vi "LB_ItemName_Tests.vi"(11 "error in":errorcluster) -> (15 "error out":errorcluster)   [LabVIEW 2016, in "DronaTest.lvlib"]
uses:
  DronaTest.lvlib
  APIs/Stimulus/ControlValue/SetValueAuto.vi
  APIs/Stimulus/ControlValue/Controls/Listbox/SetValueByItemName.vi
  APIs/Assert/AssertControlValue/Equal.vi
  <vilib>/addons/_JKI Toolkits/Caraya/classes/Assert/Assert Equal Value_Variant.vi
  <vilib>/addons/_JKI Toolkits/Caraya/classes/Assert/Assert Error.vi
  <vilib>/addons/_JKI Toolkits/Caraya/classes/Test/Test.lvclass
  Drona.lvlib
  <vilib>/SLL Toolkit/SLL Debug/SLL Debug.lvlib
  APIs/Assert/AssertControlValue/AssertControlValue.lvlib
  APIs/Stimulus/ControlValue/ControlValue.lvlib
  <vilib>/addons/_JKI Toolkits/Caraya/classes/Assert/Assert.lvclass
  APIs/Stimulus/ControlValue/Controls/Listbox/StimulusListbox.lvlib
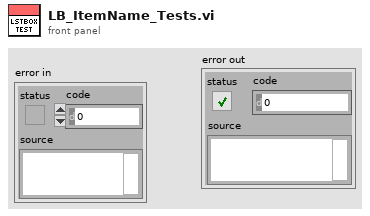
[diagram p1: front panel]
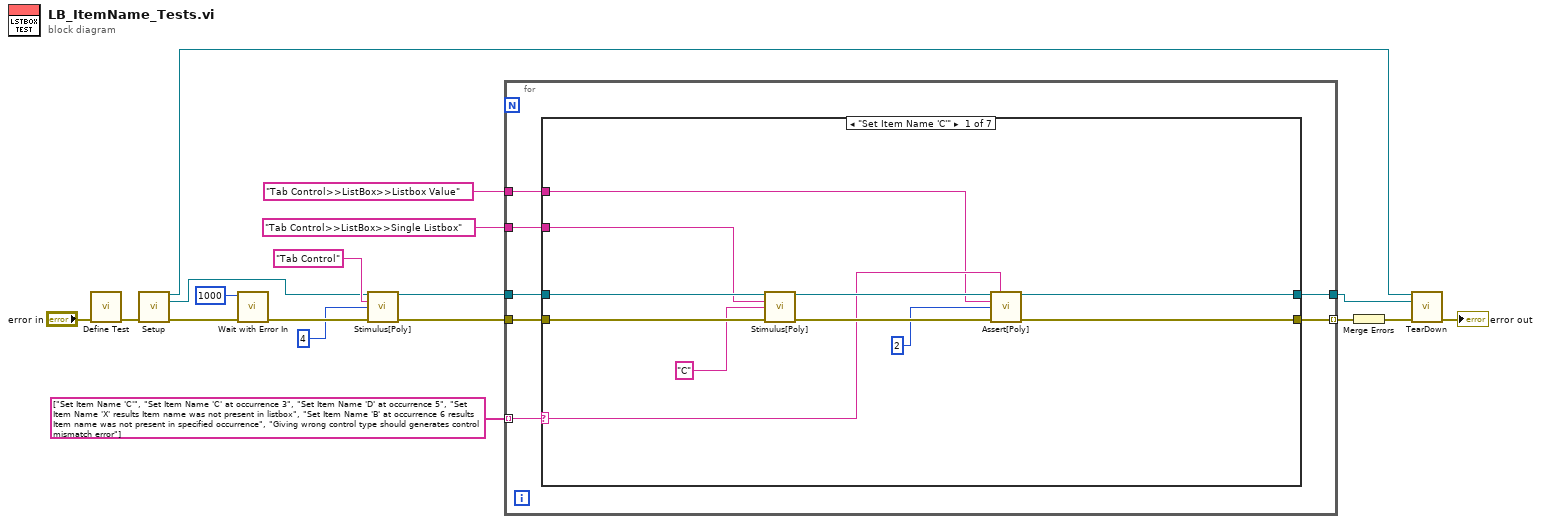
[diagram p0: block diagram]
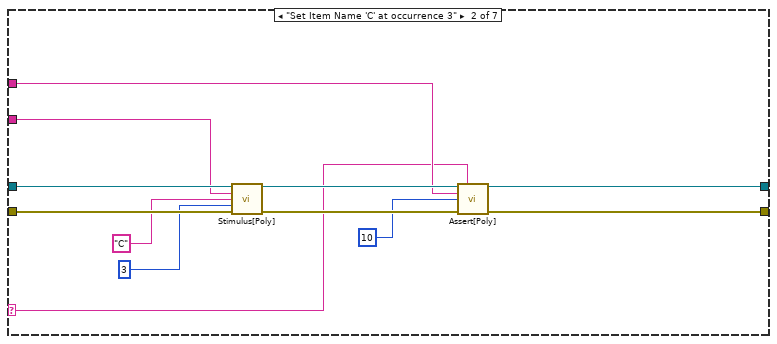
[diagram p2: hidden frame]
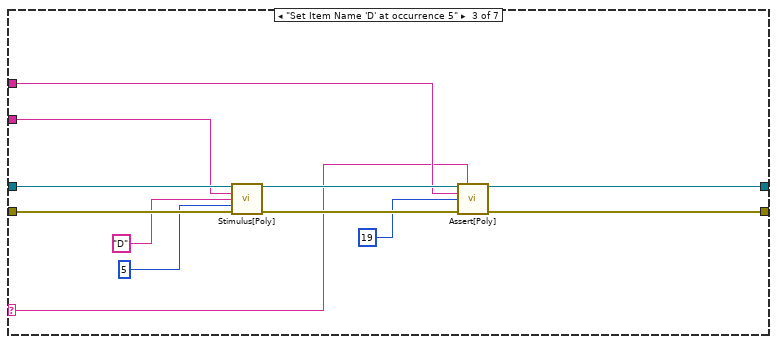
[diagram p3: hidden frame]
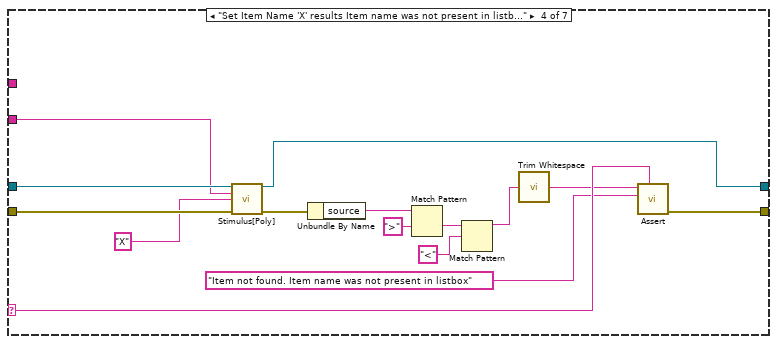
[diagram p4: hidden frame]
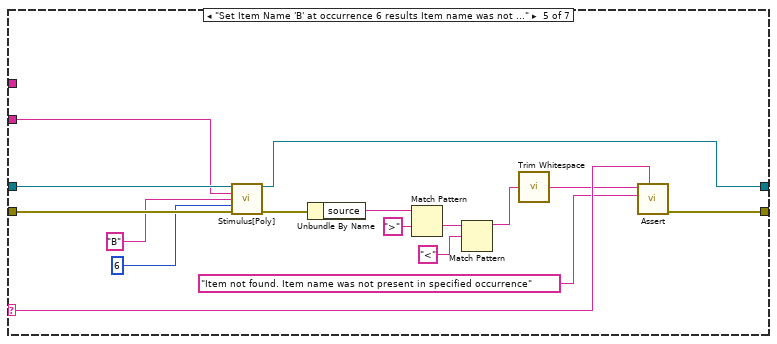
[diagram p5: hidden frame]
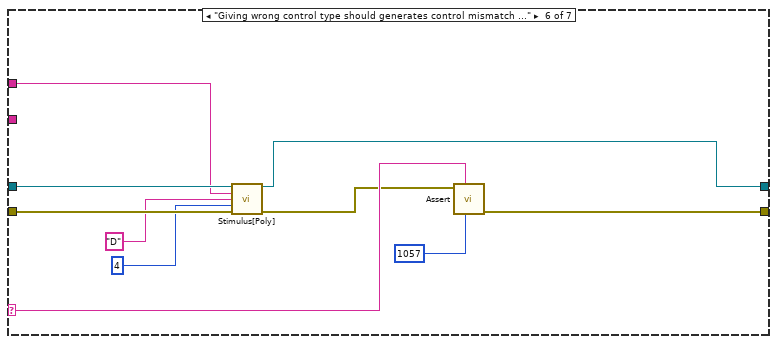
[diagram p6: hidden frame]
diagram:
  n1 = call <vilib>:"Define Test.vi"("error in (no error)"="error in") -> ("error out"=w7:errorcluster)  [unwired: 10 in]
  n2 = call "Setup.vi"("error in (no error)"=w7) -> ("Application Ref"=w2:refnum<vi>, "VI out"=w6:refnum<vi>, "error out"=w5:errorcluster)  [unwired: 12 in]
  n3 = call <vilib>:"Wait with Error In.vi"("error in (no error)"=w5, "milliseconds to wait"=u32 1000) -> ("error out"=w16:errorcluster)  [unwired: 9 in]
  n4 = call-poly "Stimulus[Poly].vi"("VI Reference In"=w6, "Control Path"="Tab Control", "Value (Signaling)"=4, "error in"=w16) -> ("VI Reference Out"=w12:refnum<vi>, "error out"=w15:errorcluster)  [unwired: 10 in]
  n5 = for {
    tunnel: w12 -> [w24]
    tunnel: "Tab Control>>ListBox>>Single Listbox" ("Control Path") -> [w23]
    tunnel: "Tab Control>>ListBox>>Listbox Value" ("Control Path") -> [w22]
    tunnel: string[] ["Set Item Name 'C'", "Set Item Name 'C' at occurrence 3", "Set Item Name 'D' at occurrence 5", "Set Item Name 'X' results Item name was not present in listbox", "Set Item Name 'B' at occurrence 6 results Item name was not present in specified occurrence", "Giving wrong control type should generates control mismatch error"] -> [w20] mode=indexing
    tunnel: [w19] -> w3
    tunnel: w15 -> [w25]
    tunnel: [w21] -> w8 mode=indexing
    n6 = case shown="\"Set Item Name 'C'\"" w20 {
      selector: w20 -> [w30 w40 w52 w71 w87 w98 _]
      tunnel: w25 -> [w36 w48 w60 w75 w91 w101 w103]
      tunnel: w24 -> [w35 w47 w59 w74 w90 w100 w102]
      tunnel: w23 -> [w26 w44 w56 w73 w89 _ _]
      tunnel: w22 -> [w27 w43 w55 _ _ w92 _]
      tunnel: [w32 w42 w54 w72 w88 w99 w103] -> w21
      tunnel: [w31 w41 w53 w70 w86 w97 w102] -> w19
      frame "Set Item Name 'C'" {
        n7 = call-poly "Stimulus[Poly].vi"("VI Reference In"=w35, "Control Path"=w26, "Item Name"="C", "Error In"=w36) -> ("VI Reference Out"=w33:refnum<vi>, "Error Out"=w34:errorcluster)  [unwired: 10 in]
        n8 = call-poly "Assert[Poly].vi"("VI Reference In"=w33, "Test Label"=w30, "Control Path"=w27, "Control Value"=2, "Error In"=w34) -> ("VI Reference Out"=w31:refnum<vi>, "Error Out"=w32:errorcluster)  [unwired: 8 in, 1 out]
      }
      frame "Set Item Name 'C' at occurrence 3" {
        n9 = call-poly "Stimulus[Poly].vi"("VI Reference In"=w47, "Control Path"=w44, "Item Name"="C", "Occurrence"=3, "Error In"=w48) -> ("VI Reference Out"=w45:refnum<vi>, "Error Out"=w46:errorcluster)  [unwired: 9 in]
        n10 = call-poly "Assert[Poly].vi"("VI Reference In"=w45, "Test Label"=w40, "Control Path"=w43, "Control Value"=10, "Error In"=w46) -> ("VI Reference Out"=w41:refnum<vi>, "Error Out"=w42:errorcluster)  [unwired: 8 in, 1 out]
      }
      frame "Set Item Name 'D' at occurrence 5" {
        n11 = call-poly "Stimulus[Poly].vi"("VI Reference In"=w59, "Control Path"=w56, "Item Name"="D", "Occurrence"=5, "Error In"=w60) -> ("VI Reference Out"=w57:refnum<vi>, "Error Out"=w58:errorcluster)  [unwired: 9 in]
        n12 = call-poly "Assert[Poly].vi"("VI Reference In"=w57, "Test Label"=w52, "Control Path"=w55, "Control Value"=19, "Error In"=w58) -> ("VI Reference Out"=w53:refnum<vi>, "Error Out"=w54:errorcluster)  [unwired: 8 in, 1 out]
      }
      frame "Set Item Name 'X' results Item name was not present in listbox" {
        n13 = call-poly "Stimulus[Poly].vi"("VI Reference In"=w74, "Control Path"=w73, "Item Name"="X", "Error In"=w75) -> ("VI Reference Out"=w70:refnum<vi>, "Error Out"=w68:errorcluster)  [unwired: 10 in]
        n14 = Unbundle By Name(w68) -> ("source"=w66:string)
        n15 = Match Pattern(string=w66, regular expression=">") -> (after substring=w64:string)  [unwired: 1 in, 3 out]
        n16 = Match Pattern(string=w64, regular expression="<") -> (before substring=w62:string)  [unwired: 1 in, 3 out]
        n17 = call <vilib>:"Trim Whitespace.vi"("string"=w62) -> ("trimmed string"=w61:string)  [unwired: 1 in]
        n18 = call-poly <vilib>:"Assert.vi"("Label"=w71, "Y"="Item not found. Item name was not present in listbox", "X"=w61) -> ("error out"=w72:errorcluster)  [unwired: 8 in]
      }
      frame "Set Item Name 'B' at occurrence 6 results Item name was not present in specified occurrence" {
        n19 = call-poly "Stimulus[Poly].vi"("VI Reference In"=w90, "Control Path"=w89, "Item Name"="B", "Occurrence"=6, "Error In"=w91) -> ("VI Reference Out"=w86:refnum<vi>, "Error Out"=w84:errorcluster)  [unwired: 9 in]
        n20 = Unbundle By Name(w84) -> ("source"=w82:string)
        n21 = Match Pattern(string=w82, regular expression=">") -> (after substring=w80:string)  [unwired: 1 in, 3 out]
        n22 = Match Pattern(string=w80, regular expression="<") -> (before substring=w78:string)  [unwired: 1 in, 3 out]
        n23 = call <vilib>:"Trim Whitespace.vi"("string"=w78) -> ("trimmed string"=w77:string)  [unwired: 1 in]
        n24 = call-poly <vilib>:"Assert.vi"("Label"=w87, "Y"="Item not found. Item name was not present in specified occurrence", "X"=w77) -> ("error out"=w88:errorcluster)  [unwired: 8 in]
      }
      frame "Giving wrong control type should generates control mismatch error" {
        n25 = call-poly "Stimulus[Poly].vi"("VI Reference In"=w100, "Control Path"=w92, "Item Name"="D", "Occurrence"=4, "Error In"=w101) -> ("VI Reference Out"=w97:refnum<vi>, "Error Out"=w94:errorcluster)  [unwired: 9 in]
        n26 = call-poly <vilib>:"Assert.vi"("error code (1)"=1057, "Label"=w98, "Error?"=w94) -> ("error out"=w99:errorcluster)  [unwired: 8 in]
      }
      frame Default {
      }
    }
  }
  n27 = Merge Errors(w8) -> (w4:errorcluster)
  n28 = call "TearDown.vi"("Application Ref"=w2, "VI in"=w3, "error in (no error)"=w4) -> ("error out"=→"error out":errorcluster)  [unwired: 12 in]
